vi "PPR-simulate-dashboard.vi"() -> ()   [LabVIEW 2019]
uses:
  <vilib>/Rock Robotics/WPI/ThirdParty/JAS_Junk/TrajLib/TypeDef/POSE2D.ctl
  <vilib>/Rock Robotics/WPI/ThirdParty/JAS_Junk/TrajLib/TypeDef/TRANSLATION2D.ctl
  <vilib>/Rock Robotics/WPI/ThirdParty/JAS_Junk/TrajLib/TypeDef/ROTATION2D.ctl
  <vilib>/Rock Robotics/WPI/ThirdParty/MJansen/PathPlanner/TypeDef/PathPlannerTrajectory.ctl
  <vilib>/Rock Robotics/WPI/ThirdParty/MJansen/PathPlanner/TypeDef/PathPlannerTrajectoryState.ctl
  <vilib>/Rock Robotics/WPI/ThirdParty/MJansen/PathPlanner/TypeDef/PathPlannerPathConstraints.ctl
  Diff_Drive_System/PPR_DRIVE_GLOBALS.vi
  Simulation/PPR_SIM_SIM_Globals.vi
  Trajectory Following/PPR_TRAJECTORY_GLOBALS.vi
  Vision_Interface/PPR_Vision_Globals.vi
  <vilib>/Rock Robotics/WPI/ThirdParty/MJansen/PathPlanner/PathPlanner24.lvlib
  <vilib>/Rock Robotics/WPI/ThirdParty/JAS_Junk/TrajLib/Trajectory_Library.lvlib
panel:
  in  "Tab Control":T1(tab)
  out "Battery Voltage":dbl(graph)
  out "Drive Speed":cluster{"Motor Dmd":dbl, "Motor Dmd":dbl}(graph)
  out "Drive Motor Demands":cluster{"Motor Dmd":dbl, "Motor Dmd":dbl}(graph)
  out "GyroReading_Degreees":dbl format="%15.3f"
  out "Encoder Distances":dbl[](array[numeric]) format="%17.2f"
  out "Encoder Velocities":dbl[](array[numeric]) format="%17.2f"
  out "Motor Demands":dbl[](array[numeric]) format="%17.2f"
  out "Battery Volts":dbl format="%16.2f"
  out "Diff Module Devices":T2(array[cluster])
  out "Wheel \nSpeed Dmd":dbl[](array[numeric]) format="%17.3f"
  out "Diff Drive Motor output":T3(graph)
  out "Diff Drive Speed M/S":T4(graph)
  out "Diff Drive Speed Error  M/S":T5(graph)
  out "Closed Loop Control":bool
  out "Orientation Angle Dmd_Rad":dbl format="%17.3f"
  out "GyroHeading_Radians":dbl format="%17.2f"
  out "Orientation Angle Error_Rad":dbl format="%17.3f"
  out "Orientation Correct CO":dbl format="%17.3f"
  out "Wheel Out":dbl[](array[numeric]) format="%17.3f"
  out "Wheel \nSpeed M/S":dbl[](array[numeric]) format="%17.3f"
  out "Wheel Speed Err":dbl[](array[numeric]) format="%17.3f"
  out "Limited Wheel \nSpeed Dmd":dbl[](array[numeric]) format="%17.3f"
  out "Sim ABS Pose":T6={"TRANSLATION"={"X"=0.0, "Y"=0.0}, "ROTATION"={"VALUE"=0.0, "COS"=1.0, "SIN"=0.0}} {"ROTATION"."SIN" format="%13.4f"; "ROTATION"."COS" format="%13.4f"; "ROTATION"."VALUE" format="%13.4f"; "TRANSLATION"."Y" format="%14.3f"; "TRANSLATION"."X" format="%14.3f"}
  out "Traj Heading Err DEG":dbl format="%17.2f"
  out "Traj Pos Err Ft":dbl format="%17.2f"
  out "Traj Y Err Ft":dbl format="%17.2f"
  out "Traj X Err Ft":dbl format="%17.2f"
  out "Vision Pose":T6={"TRANSLATION"={"X"=0.0, "Y"=0.0}, "ROTATION"={"VALUE"=0.0, "COS"=1.0, "SIN"=0.0}} {"ROTATION"."SIN" format="%13.4f"; "ROTATION"."COS" format="%13.4f"; "ROTATION"."VALUE" format="%13.4f"; "TRANSLATION"."Y" format="%14.3f"; "TRANSLATION"."X" format="%14.3f"}
  out "Vision\nPose":bool
  out "Trajectory Status":T9(graph)
  out "Trajectory Execution \nClosed Loop":bool
  out "Trajectory Error":T10(graph)
  out "Traj_OnTarget":bool
  out "Traj Heading Dmd Deg":dbl format="%17.2f"
  out "Traj Final Heading Dmd Deg":dbl format="%17.2f"
  out "Traj Sample Time Sec":dbl format="%17.2f"
  out "Traj Rot Vel FF Rad/Sec":dbl format="%17.2f"
  out "Relative Trajectory Pose":T6={"TRANSLATION"={"X"=0.0, "Y"=0.0}, "ROTATION"={"VALUE"=0.0, "COS"=1.0, "SIN"=0.0}} {"ROTATION"."SIN" format="%13.4f"; "ROTATION"."COS" format="%13.4f"; "ROTATION"."VALUE" format="%13.4f"; "TRANSLATION"."Y" format="%14.3f"; "TRANSLATION"."X" format="%14.3f"}
  out "Absolute Odometry \nPose":T6={"TRANSLATION"={"X"=0.0, "Y"=0.0}, "ROTATION"={"VALUE"=0.0, "COS"=1.0, "SIN"=0.0}} {"ROTATION"."SIN" format="%13.4f"; "ROTATION"."COS" format="%13.4f"; "ROTATION"."VALUE" format="%13.4f"; "TRANSLATION"."Y" format="%14.3f"; "TRANSLATION"."X" format="%14.3f"}
  out "Other ABS Odometry\nPose":T6={"TRANSLATION"={"X"=0.0, "Y"=0.0}, "ROTATION"={"VALUE"=0.0, "COS"=1.0, "SIN"=0.0}} {"ROTATION"."SIN" format="%13.4f"; "ROTATION"."COS" format="%13.4f"; "ROTATION"."VALUE" format="%13.4f"; "TRANSLATION"."Y" format="%14.3f"; "TRANSLATION"."X" format="%14.3f"}
  out "Absolue Trajectory":cluster{dbl[], dbl[]}(graph)
  out "Absolute Trajectory":T11 {"States"."TargetHolonomicRotation"."SIN" format="%13.4f"; "States"."TargetHolonomicRotation"."COS" format="%13.4f"; "States"."TargetHolonomicRotation"."VALUE" format="%13.4f"; "States"."Heading"."SIN" format="%13.4f"; "States"."Heading"."COS" format="%13.4f"; "States"."Heading"."VALUE" format="%13.4f"; "States"."PositionMeters"."Y" format="%14.3f"; "States"."PositionMeters"."X" format="%14.3f"}
  out "Relative Trajectory":cluster{dbl[], dbl[]}(graph)
  # "SIMULATION"
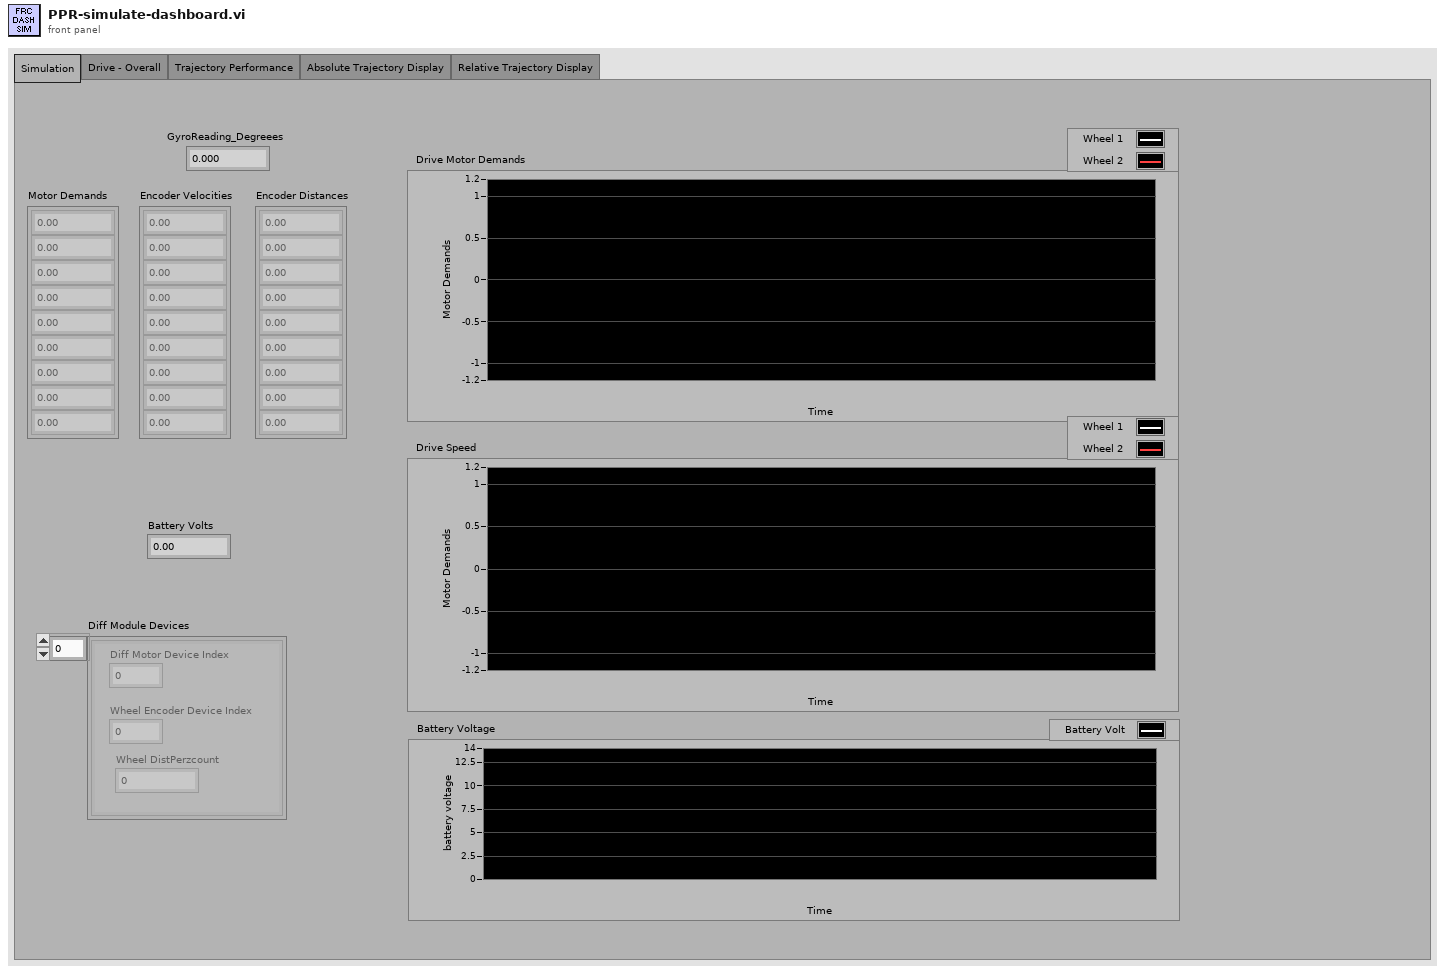
[diagram p1: front panel]
types:
  T1 = enum32{"Simulation", "Drive - Overall", "Trajectory Performance", "Absolute Trajectory Display", "Relative Trajectory Display"}
  T2 = cluster{"Diff Motor Device Index":i32, "Wheel Encoder Device Index":i32, "Wheel DistPerzcount":dbl}[]
  T3 = cluster{"Left Wheel Motor Out":dbl, "Right Wheel Motor Out":dbl}
  T4 = cluster{"Left Wheel Speed M/S":dbl, "Right Wheel Speed M/S":dbl}
  T5 = cluster{"Left Wheel Speed Err M/S":dbl, "Right Wheel Speed Err M/S":dbl}
  T6 = typedef "Trajectory_Library.lvlib/POSE2D.ctl" = cluster{"TRANSLATION":T7, "ROTATION":T8}
  T7 = typedef "Trajectory_Library.lvlib/TRANSLATION2D.ctl" = cluster{"X":dbl, "Y":dbl}
  T8 = typedef "Trajectory_Library.lvlib/ROTATION2D.ctl" = cluster{"VALUE":dbl, "COS":dbl, "SIN":dbl}
  T9 = cluster{dbl, dbl, dbl, "Traj_Sample_Time_Sec":dbl}
  T10 = cluster{"Traj X Err":dbl, "Traj Y Err":dbl, "Traj Heading Err":dbl}
  T11 = typedef "PathPlanner24.lvlib/PathPlannerTrajectory.ctl" = cluster{"States":T12[]}
  T12 = typedef "PathPlanner24.lvlib/PathPlannerTrajectoryState.ctl" = cluster{"TimeSeconds":dbl, "VelocityMPS":dbl, "AccerationMpsSq":dbl, "HeadingAngularVelRadPerSec":dbl, "PositionMeters":T7, "Heading":T8, "TargetHolonomicRotation":T8, "CurvatureRadPerMeter":dbl, "PathPlannerConstraints":T13, "DeltaPos":dbl}
  T13 = typedef "PathPlanner24.lvlib/PathPlannerPathConstraints.ctl" = cluster{"MaxVelocityMps;":dbl, "MaxAccelerationMpsSq;":dbl, "MaxAngularVelRadPsEc;":dbl, "MaxAngularAccRadPSecSq":dbl, "Exists":bool, "Unlimited":bool, "NominalVoltageVolts":dbl}
  T14 = cluster{"Traj X Err_FT":dbl, "Traj Y Err_FT":dbl, "Traj Heading Err_DEG":dbl}
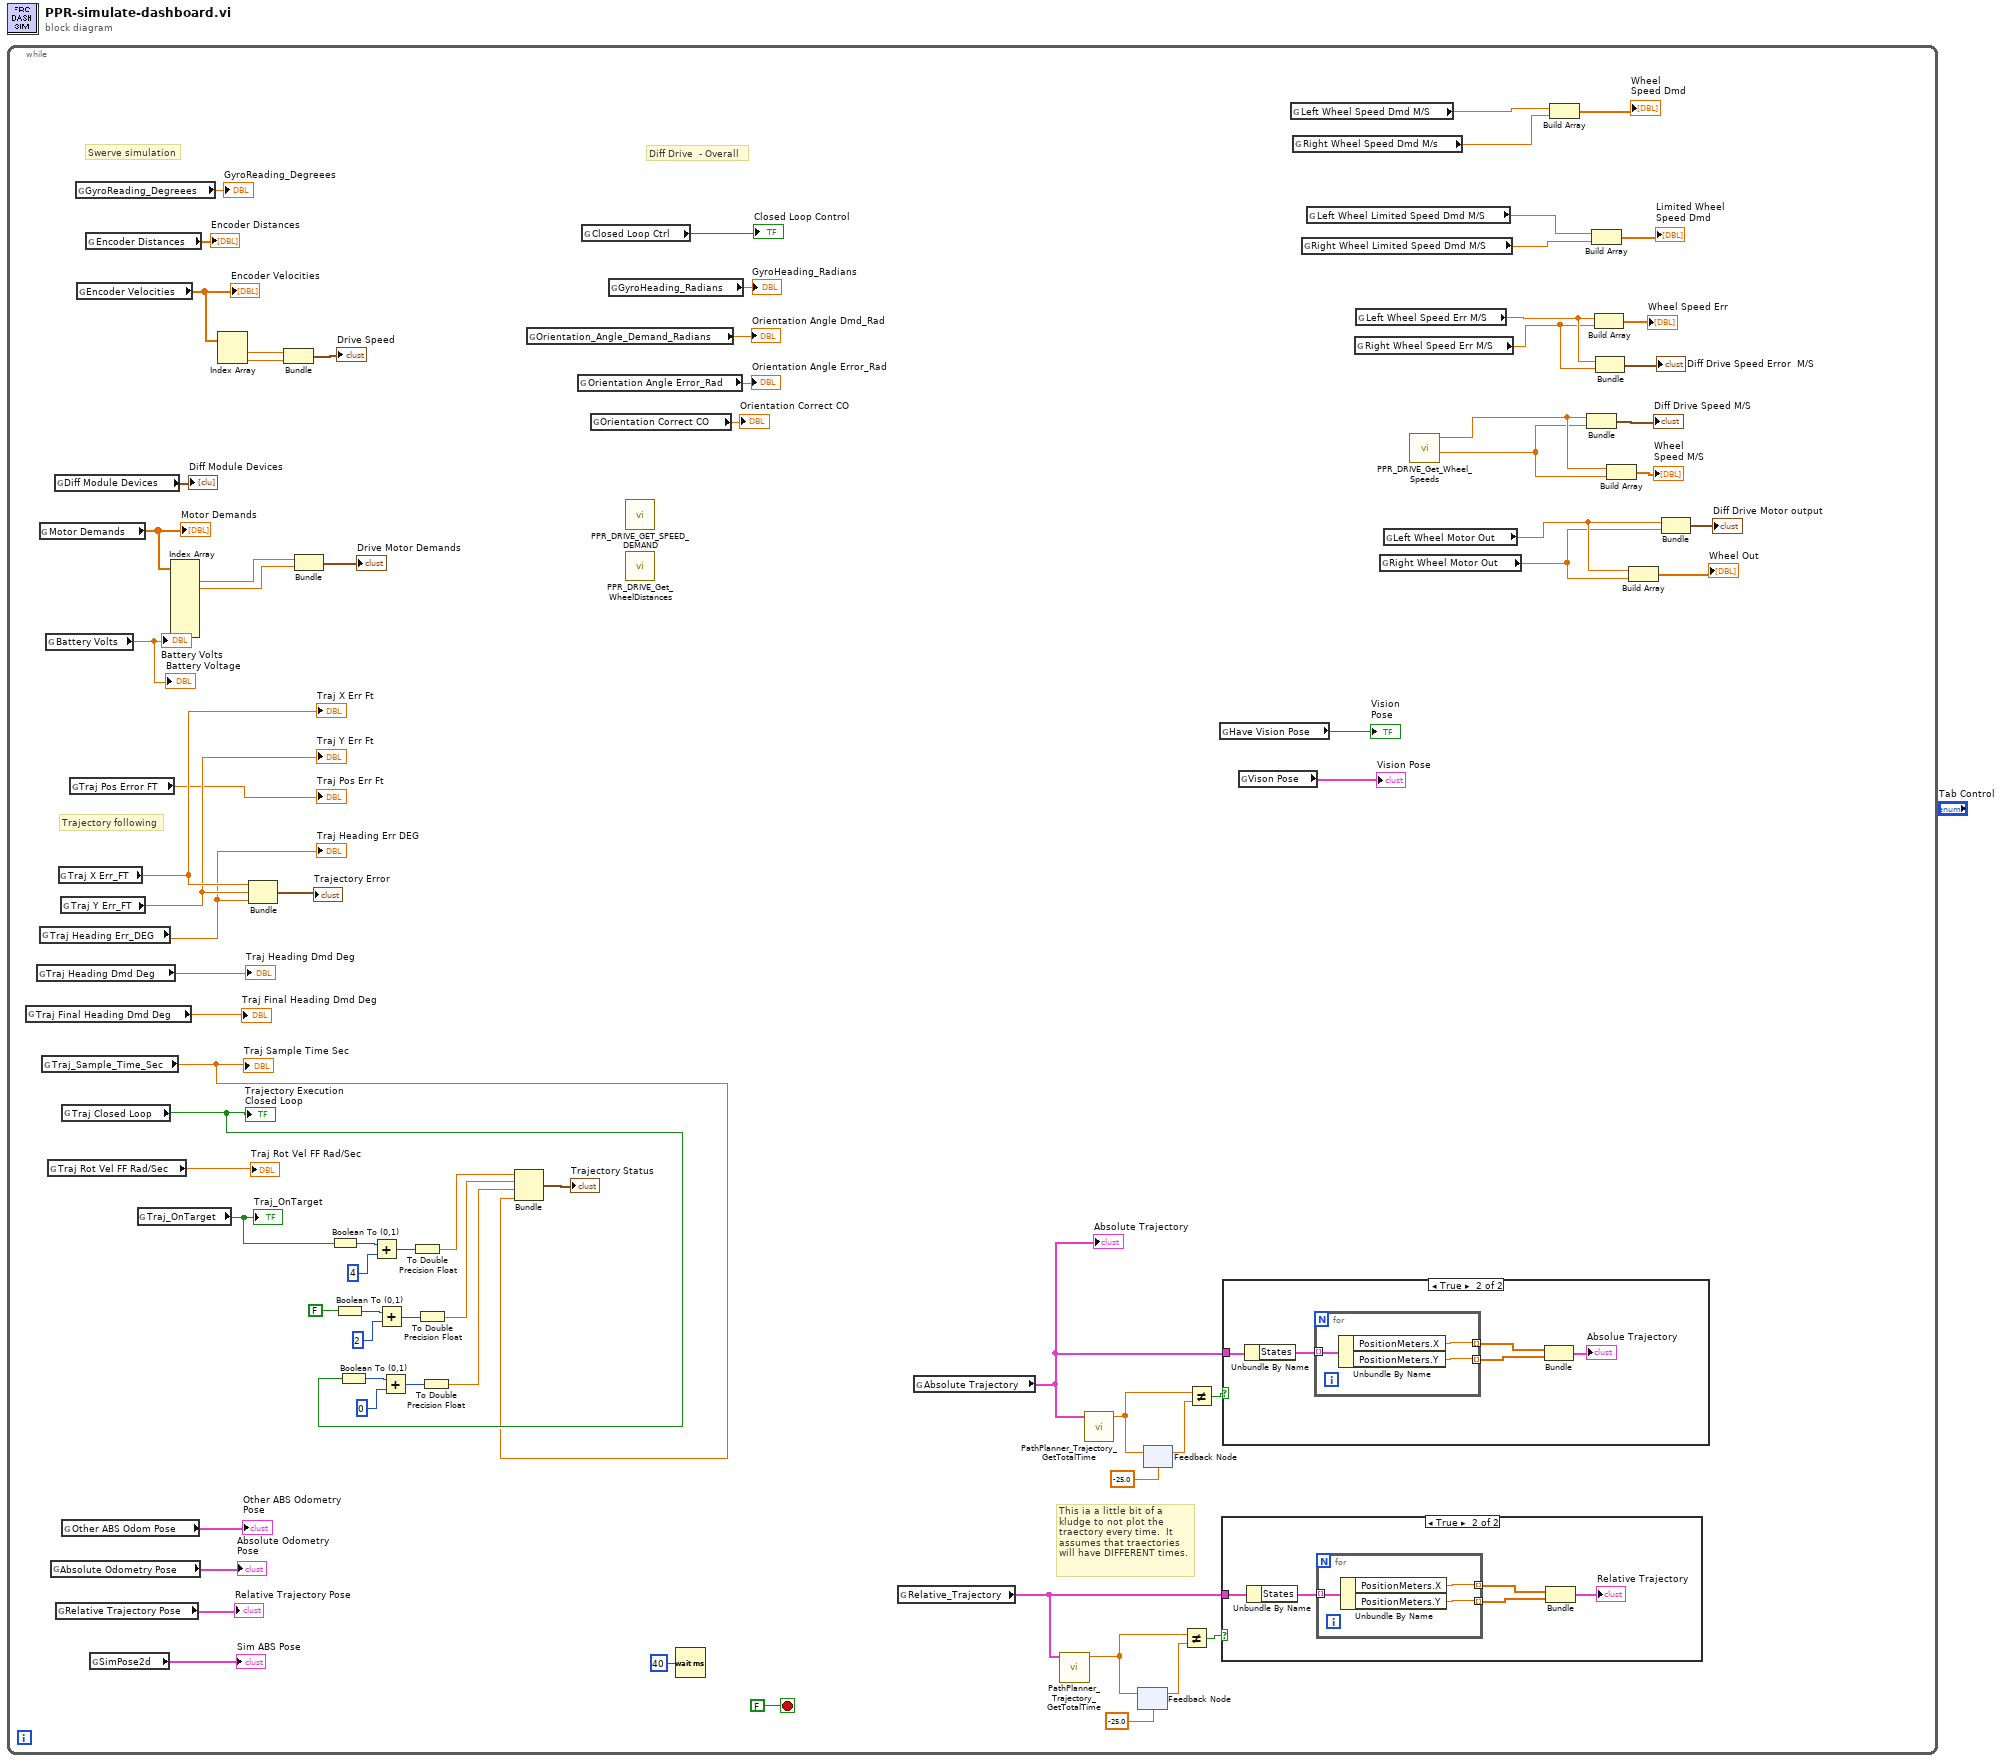
[diagram p0: block diagram]
diagram:
  n1 = while {
    stop <- FALSE stop-if-true
    # "This ia a little bit of a \nkludge to not plot the\ntraectory every time.  It \nassumes that traectories\nwill have DIFFERENT times."
    # "Trajectory following"
    # "Swerve simulation"
    # "Diff Drive  - Overall"
    n2 = global read "PPR_TRAJECTORY_GLOBALS.vi" "Traj Final Heading Dmd Deg"() -> (→"Traj Final Heading Dmd Deg":dbl)
    n3 = global read "PPR_TRAJECTORY_GLOBALS.vi" "Traj Heading Dmd Deg"() -> (→"Traj Heading Dmd Deg":dbl)
    n4 = global read "PPR_SIM_SIM_Globals.vi" "Motor Demands"() -> (w69:dbl[])
    "Motor Demands" <- w69
    n5 = global read "PPR_TRAJECTORY_GLOBALS.vi" "Traj Heading Err_DEG"() -> (w3:dbl)
    "Traj Heading Err DEG" <- w3
    n6 = global read "PPR_TRAJECTORY_GLOBALS.vi" "Traj_Sample_Time_Sec"() -> (w48:dbl)
    "Traj Sample Time Sec" <- w48
    n7 = global read "PPR_SIM_SIM_Globals.vi" "Battery Volts"() -> (→"Battery Volts" →"Battery Voltage":dbl)
    n8 = global read "PPR_TRAJECTORY_GLOBALS.vi" "Traj Rot Vel FF Rad/Sec"() -> (→"Traj Rot Vel FF Rad/Sec":dbl)
    n9 = global read "PPR_TRAJECTORY_GLOBALS.vi" "Absolute Odometry Pose"() -> (→"Absolute Odometry \nPose":T6)
    n10 = global read "PPR_SIM_SIM_Globals.vi" "Diff Module Devices"() -> (→"Diff Module Devices":T2)
    n11 = global read "PPR_TRAJECTORY_GLOBALS.vi" "Relative Trajectory Pose"() -> (→"Relative Trajectory Pose":T6)
    n12 = global read "PPR_TRAJECTORY_GLOBALS.vi" "Traj X Err_FT"() -> (w5:dbl)
    "Traj X Err Ft" <- w5
    n13 = global read "PPR_TRAJECTORY_GLOBALS.vi" "Traj Y Err_FT"() -> (w4:dbl)
    "Traj Y Err Ft" <- w4
    n14 = global read "PPR_TRAJECTORY_GLOBALS.vi" "Traj Closed Loop"() -> (w50:bool)
    "Trajectory Execution \nClosed Loop" <- w50
    n15 = global read "PPR_TRAJECTORY_GLOBALS.vi" "Other ABS Odom Pose"() -> (→"Other ABS Odometry\nPose":T6)
    n16 = global read "PPR_TRAJECTORY_GLOBALS.vi" "Traj Pos Error FT"() -> (→"Traj Pos Err Ft":dbl)
    n17 = global read "PPR_SIM_SIM_Globals.vi" "GyroReading_Degreees"() -> (→"GyroReading_Degreees":dbl)
    n18 = global read "PPR_SIM_SIM_Globals.vi" "Encoder Velocities"() -> (w9:dbl[])
    "Encoder Velocities" <- w9
    n19 = global read "PPR_SIM_SIM_Globals.vi" "Encoder Distances"() -> (→"Encoder Distances":dbl[])
    n20 = global read "PPR_SIM_SIM_Globals.vi" "SimPose2d"() -> (→"Sim ABS Pose":T6)
    n21 = global read "PPR_TRAJECTORY_GLOBALS.vi" "Traj_OnTarget"() -> (w62:bool)
    "Traj_OnTarget" <- w62
    n22 = Index Array(array=w69) -> (element #1=w68:dbl, element #2=w10:dbl)  [unwired: 8 in, 6 out]
    n23 = Index Array(array=w9) -> (element #1=w8:dbl, element #2=w7:dbl)  [unwired: 2 in]
    n24 = Bundle("Traj X Err_FT"=w5, "Traj Y Err_FT"=w4, "Traj Heading Err_DEG"=w3) -> (→"Trajectory Error":T14)  [unwired: 1 in]
    n25 = Bundle("Motor Dmd"=w8, "Motor Dmd"=w7) -> (→"Drive Speed":cluster{"Motor Dmd":dbl, "Motor Dmd":dbl})  [unwired: 1 in]
    n26 = Bundle("Motor Dmd"=w68, "Motor Dmd"=w10) -> (→"Drive Motor Demands":cluster{"Motor Dmd":dbl, "Motor Dmd":dbl})  [unwired: 1 in]
    n27 = Boolean To (0,1)(Boolean=w62) -> (0, 1=w60:i16)
    n28 = Boolean To (0,1)(Boolean=FALSE) -> (0, 1=w57:i16)
    n29 = Boolean To (0,1)(Boolean=w50) -> (0, 1=w53:i16)
    n30 = Add(x=w60, y=i16 4) -> (x+y=w59:i16)
    n31 = Add(x=w57, y=i16 2) -> (x+y=w56:i16)
    n32 = Add(x=w53, y=i16 0) -> (x+y=w52:i16)
    n33 = To Double Precision Float(number=w59) -> (double precision float=w61:dbl)
    n34 = To Double Precision Float(number=w56) -> (double precision float=w54:dbl)
    n35 = To Double Precision Float(number=w52) -> (double precision float=w49:dbl)
    n36 = Bundle(w61, w54, w49, "Traj_Sample_Time_Sec"=w48) -> (→"Trajectory Status":T9)  [unwired: 1 in]
    n37 = global read "PPR_DRIVE_GLOBALS.vi" "Orientation_Angle_Demand_Radians"() -> (→"Orientation Angle Dmd_Rad":dbl)
    n38 = global read "PPR_DRIVE_GLOBALS.vi" "Orientation Angle Error_Rad"() -> (→"Orientation Angle Error_Rad":dbl)
    n39 = global read "PPR_DRIVE_GLOBALS.vi" "Closed Loop Ctrl"() -> (→"Closed Loop Control":bool)
    n40 = global read "PPR_DRIVE_GLOBALS.vi" "Orientation Correct CO"() -> (→"Orientation Correct CO":dbl)
    n41 = global read "PPR_DRIVE_GLOBALS.vi" "GyroHeading_Radians"() -> (→"GyroHeading_Radians":dbl)
    n42 = call "PPR_DRIVE_GET_SPEED_DEMAND.vi"() -> ()  [unwired: 10 in, 2 out]
    n43 = call "PPR_DRIVE_Get_WheelDistances.vi"() -> ()  [unwired: 10 in, 2 out]
    n44 = Wait (ms)(milliseconds to wait=u32 40) -> ()  [unwired: 1 out]
    n45 = global read "PPR_TRAJECTORY_GLOBALS.vi" "Relative_Trajectory"() -> (w30:T11)
    n46 = global read "PPR_TRAJECTORY_GLOBALS.vi" "Absolute Trajectory"() -> (w32:T11)
    "Absolute Trajectory" <- w32
    n47 = call <vilib>:"PathPlanner_Trajectory_GetTotalTime.vi"("PathPlannerTrajectory"=w30) -> ("TotalTimeSeconds"=w29:dbl)  [unwired: 10 in]
    n48 = call <vilib>:"PathPlanner_Trajectory_GetTotalTime.vi"("PathPlannerTrajectory"=w32) -> ("TotalTimeSeconds"=w31:dbl)  [unwired: 10 in]
    n49 = feedback #1(-25.0 ("TotalTime_Sec")) -> (w34:dbl)
    n50 = feedback-in #1(w29) -> ()
    n51 = feedback #2(-25.0 ("TotalTime_Sec")) -> (w37:dbl)
    n52 = feedback-in #2(w31) -> ()
    n53 = Not Equal?(x=w29, y=w34) -> (x != y?=w33:bool)
    n54 = Not Equal?(x=w31, y=w37) -> (x != y?=w36:bool)
    n55 = global read "PPR_Vision_Globals.vi" "Have Vision Pose"() -> (→"Vision\nPose":bool)
    n56 = case shown="True" w33 {
      tunnel: w30 -> [_ w80]
      frame False {
      }
      frame True {
        n57 = Unbundle By Name(w80) -> ("States"=w81:T12[])
        n58 = for {
          tunnel: [w86] -> w82 mode=indexing
          tunnel: [w85] -> w83 mode=indexing
          tunnel: w81 -> [w84] mode=indexing
          n59 = Unbundle By Name(w84) -> ("PositionMeters.X"=w86:dbl, "PositionMeters.Y"=w85:dbl)
        }
        n60 = Bundle(w82, w83) -> (→"Relative Trajectory":cluster{dbl[], dbl[]})  [unwired: 1 in]
      }
    }
    n61 = case shown="True" w36 {
      tunnel: w32 -> [_ w87]
      frame False {
      }
      frame True {
        n62 = Unbundle By Name(w87) -> ("States"=w89:T12[])
        n63 = for {
          tunnel: [w94] -> w90 mode=indexing
          tunnel: [w93] -> w91 mode=indexing
          tunnel: w89 -> [w92] mode=indexing
          n64 = Unbundle By Name(w92) -> ("PositionMeters.X"=w94:dbl, "PositionMeters.Y"=w93:dbl)
        }
        n65 = Bundle(w90, w91) -> (→"Absolue Trajectory":cluster{dbl[], dbl[]})  [unwired: 1 in]
      }
    }
    n66 = global read "PPR_Vision_Globals.vi" "Vison Pose"() -> (→"Vision Pose":T6)
    n67 = global read "PPR_DRIVE_GLOBALS.vi" "Left Wheel Speed Dmd M/S"() -> (w15:dbl)
    n68 = global read "PPR_DRIVE_GLOBALS.vi" "Right Wheel Speed Dmd M/s"() -> (w14:dbl)
    n69 = global read "PPR_DRIVE_GLOBALS.vi" "Right Wheel Limited Speed Dmd M/S"() -> (w11:dbl)
    n70 = global read "PPR_DRIVE_GLOBALS.vi" "Left Wheel Limited Speed Dmd M/S"() -> (w12:dbl)
    n71 = global read "PPR_DRIVE_GLOBALS.vi" "Right Wheel Speed Err M/S"() -> (w17:dbl)
    n72 = global read "PPR_DRIVE_GLOBALS.vi" "Left Wheel Speed Err M/S"() -> (w18:dbl)
    n73 = global read "PPR_DRIVE_GLOBALS.vi" "Right Wheel Motor Out"() -> (w23:dbl)
    n74 = global read "PPR_DRIVE_GLOBALS.vi" "Left Wheel Motor Out"() -> (w24:dbl)
    n75 = call "PPR_DRIVE_Get_Wheel_Speeds.vi"() -> ("Right Wheel Speed M/S"=w20:dbl, "Left Wheel Speed M/S"=w21:dbl)  [unwired: 10 in]
    n76 = Build Array(w15, w14) -> (→"Wheel \nSpeed Dmd":dbl[])
    n77 = Bundle("Left Wheel Speed M/S"=w21, "Right Wheel Speed M/S"=w20) -> (→"Diff Drive Speed M/S":T4)  [unwired: 1 in]
    n78 = Build Array(w12, w11) -> (→"Limited Wheel \nSpeed Dmd":dbl[])
    n79 = Build Array(w18, w17) -> (→"Wheel Speed Err":dbl[])
    n80 = Bundle("Left Wheel Speed Err M/S"=w18, "Right Wheel Speed Err M/S"=w17) -> (→"Diff Drive Speed Error  M/S":T5)  [unwired: 1 in]
    n81 = Build Array(w21, w20) -> (→"Wheel \nSpeed M/S":dbl[])
    n82 = Build Array(w24, w23) -> (→"Wheel Out":dbl[])
    n83 = Bundle("Left Wheel Motor Out"=w24, "Right Wheel Motor Out"=w23) -> (→"Diff Drive Motor output":T3)  [unwired: 1 in]
  }
